vi "Read out IMON.vi"(4 "get more?":bool, 5 "All Channels (T)":bool=TRUE, 7 "Channel":u8, 8 "error in (no error)":errorcluster, 11 "BoardHandle":T2) -> (0 "error out":errorcluster, 1 "IMon constants":T1(array[cluster]), 2 "IMon values (uA)":dbl[](array[numeric]) format="%.2f", 3 "BoardHandle out":T2)   [LabVIEW 2020, in "CAEN PSM.lvlib"]
doc: "This function returns Imon value"
uses:
  CAEN PSM.lvlib
  Private/BoardHandle.ctl
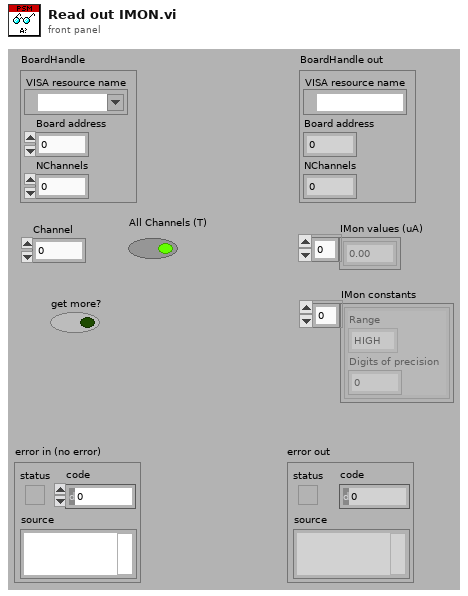
[diagram p1: front panel]
types:
  T1 = cluster{"Range":enum16{"HIGH", "LOW"}, "Digits of precision":i32}[]
  T2 = typedef "CAEN PSM.lvlib/BoardHandle.ctl" = cluster{"VISA resource name":refnum<visa-resource-name>, "Board address":i8, "NChannels":u8}
  T3 = cluster{"Range":enum16{"HIGH", "LOW"}, "Digits of precision":i32}
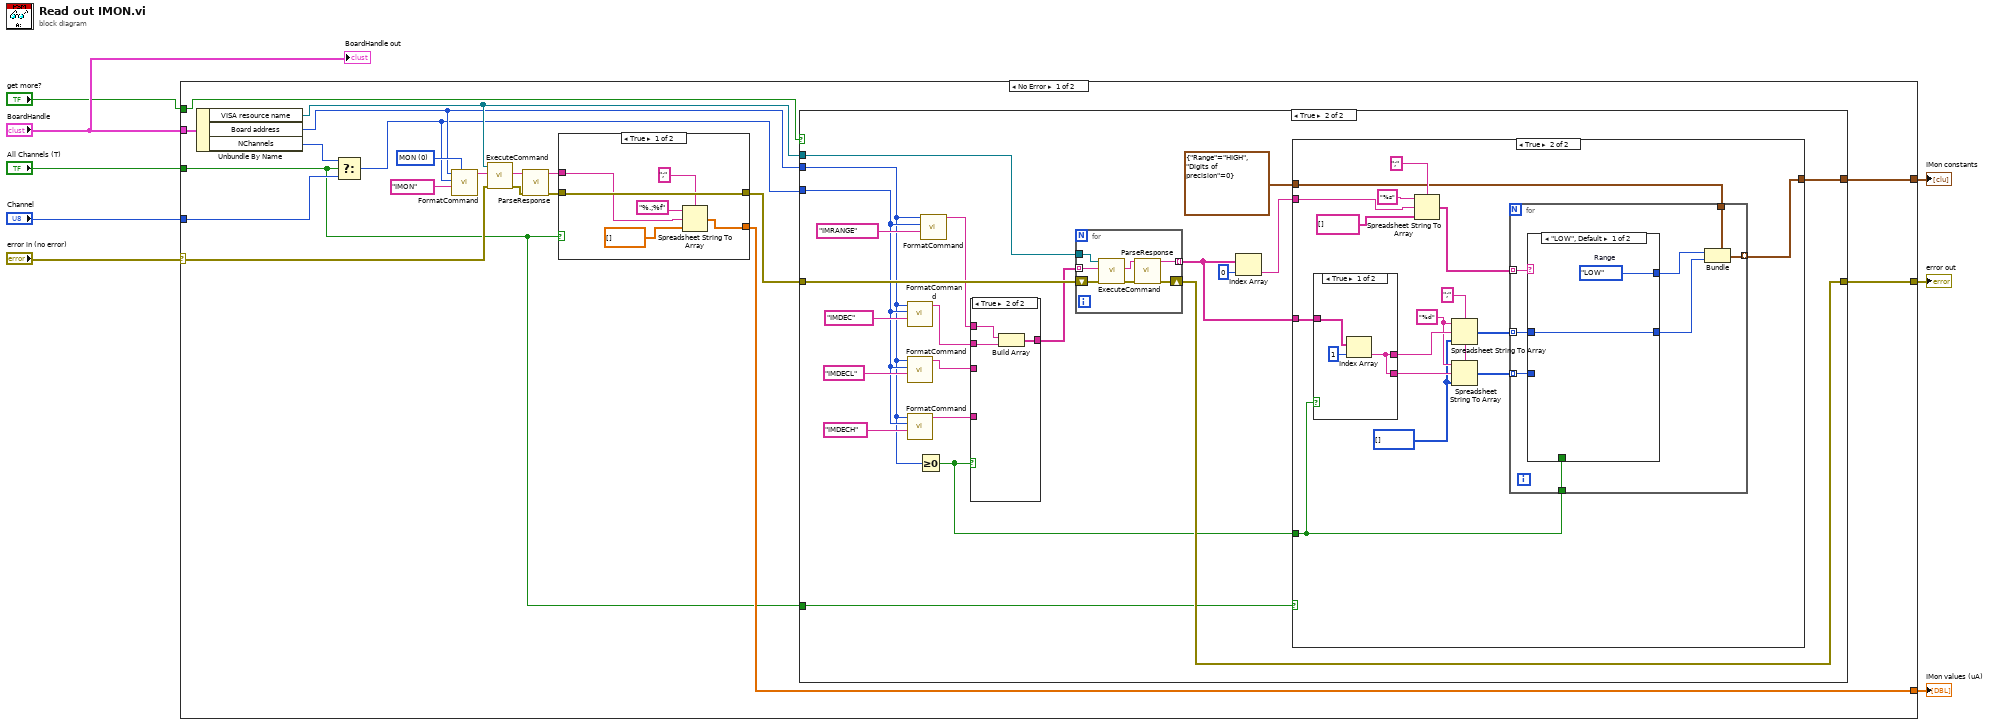
[diagram p0: block diagram]
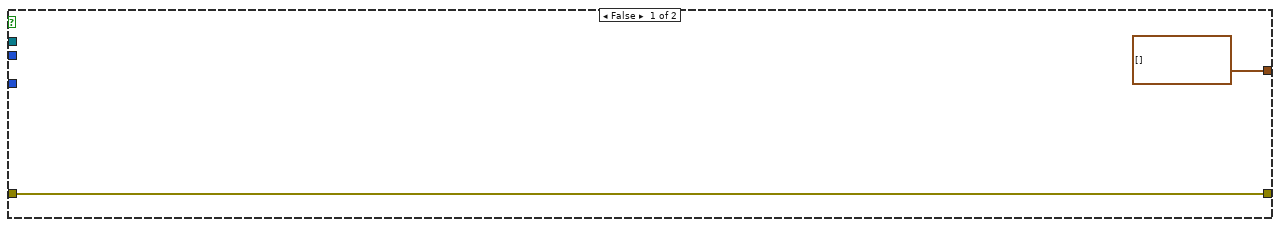
[diagram p2: hidden frame]
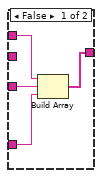
[diagram p3: hidden frame]
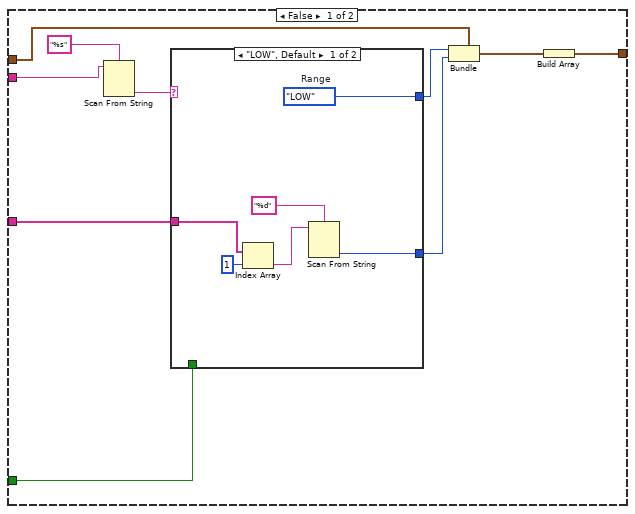
[diagram p4: hidden frame]
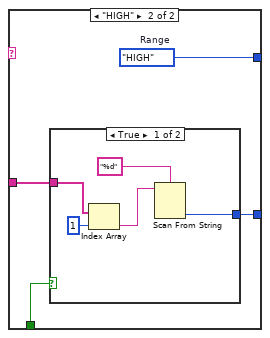
[diagram p5: hidden frame]
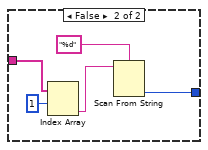
[diagram p6: hidden frame]
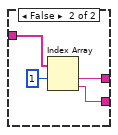
[diagram p7: hidden frame]
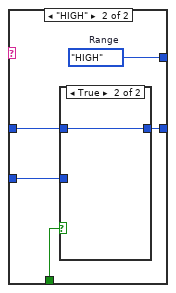
[diagram p8: hidden frame]
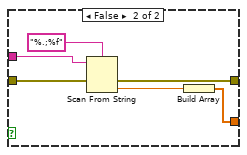
[diagram p10: hidden frame]
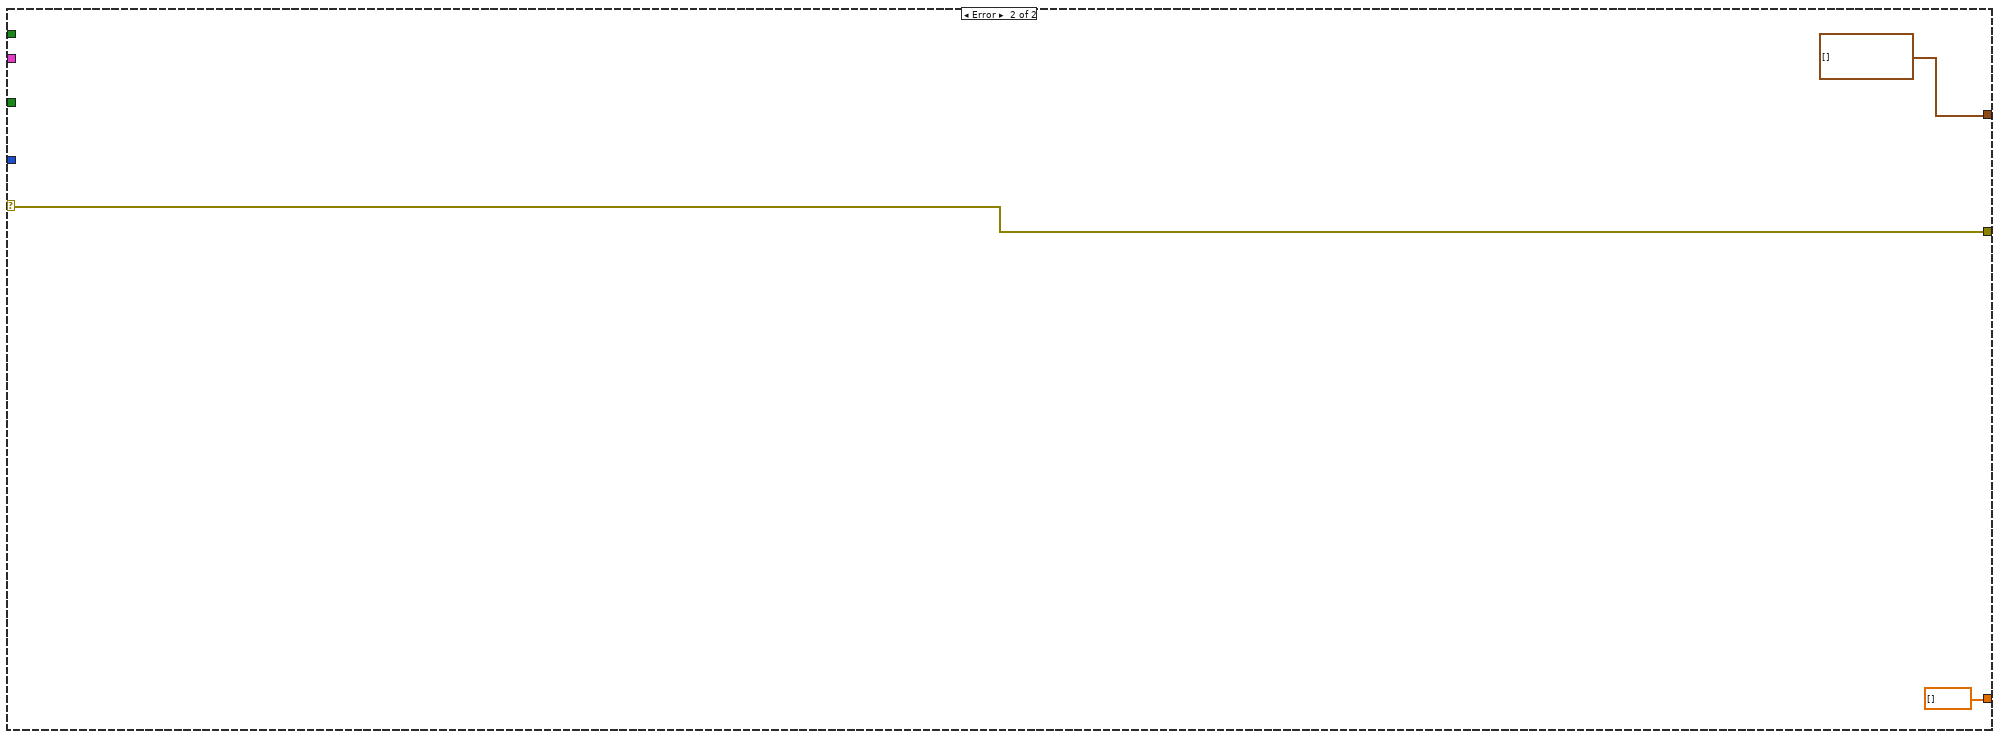
[diagram p11: hidden frame]
diagram:
  n1 = case shown="No Error" "error in (no error)" {
    selector: "error in (no error)" -> [w22 w150]
    tunnel: "All Channels (T)" -> [w9 _]
    tunnel: "Channel" -> [w27 _]
    tunnel: [w11 w150] -> w5
    tunnel: "BoardHandle" -> [w23 _]
    tunnel: [w17 dbl[] [] ("Trip value(s) s")] -> w3
    tunnel: "get more?" -> [w16 _]
    tunnel: [w10 T1 []] -> w1
    frame No Error {
      w28 = u8 0 items=["MON", "SET"] ("CMD")
      n2 = Unbundle By Name(w23) -> ("VISA resource name"=w15:refnum<visa-resource-name>, "Board address"=w14:i8, "NChannels"=w20:u8)
      n3 = Select(t=w20, s=w9, f=w27) -> (s? t:f=w13:u8)
      n4 = call "FormatCommand.vi"("CMD (MON)"=w28, "PAR"="IMON", "CH"=w13, "BD (0)"=w14) -> ("cmd"=w26:string)  [unwired: 7 in]
      n5 = call "ExecuteCommand.vi"("error in (no error)"=w22, "Command"=w26, "VISA resource name"=w15) -> ("error out"=w25:errorcluster, "Response"=w24:string)  [unwired: 6 in, 1 out]
      n6 = call "ParseResponse.vi"("error in (no error)"=w25, "Response"=w24) -> ("error out"=w18:errorcluster, "val"=w19:string)  [unwired: 6 in, 2 out]
      n7 = case shown="True" w9 {
        tunnel: w19 -> [w136 w147]
        tunnel: w18 -> [w141 w145]
        tunnel: [w141 w144] -> w12
        tunnel: [w137 w142] -> w17
        frame True {
          n8 = Spreadsheet String To Array(delimiter (Tab)=";", format string="%.;%f", spreadsheet string=w136, array type (2D Dbl)=dbl[] []) -> (array=w137:dbl[])
        }
        frame False {
          n9 = Scan From String(format string="%.;%f", input string=w147, error in=w145) -> (error out=w144:errorcluster, output 1=w143:dbl)  [unwired: 2 in, 2 out]
          n10 = Build Array(w143) -> (w142:dbl[])
        }
      }
      n11 = case shown="True" w16 {
        tunnel: w12 -> [w30 w48]
        tunnel: [w30 w47] -> w11
        tunnel: w15 -> [_ w49]
        tunnel: w14 -> [_ w35]
        tunnel: w13 -> [_ w41]
        tunnel: [T1 [] w45] -> w10
        tunnel: w9 -> [_ w44]
        frame False {
        }
        frame True {
          n12 = call "FormatCommand.vi"("PAR"="IMDEC", "CH"=w41, "BD (0)"=w35) -> ("cmd"=w40:string)  [unwired: 8 in]
          n13 = call "FormatCommand.vi"("PAR"="IMDECL", "CH"=w41, "BD (0)"=w35) -> ("cmd"=w37:string)  [unwired: 8 in]
          n14 = call "FormatCommand.vi"("PAR"="IMDECH", "CH"=w41, "BD (0)"=w35) -> ("cmd"=w36:string)  [unwired: 8 in]
          n15 = Greater Or Equal To 0?(x=w35) -> (x >= 0?=w32:bool)
          n16 = call "FormatCommand.vi"("PAR"="IMRANGE", "CH"=w41, "BD (0)"=w35) -> ("cmd"=w39:string)  [unwired: 8 in]
          n17 = case shown="True" w32 {
            tunnel: w40 -> [_ w58]
            tunnel: w39 -> [w55 w57]
            tunnel: [w52 w56] -> w38
            tunnel: w37 -> [w54 _]
            tunnel: w36 -> [w53 _]
            frame False {
              n18 = Build Array(w55, w54, w53) -> (w52:string[])
            }
            frame True {
              n19 = Build Array(w57, w58) -> (w56:string[])
            }
          }
          n20 = for {
            tunnel: w38 -> [w135] mode=indexing
            tunnel: w49 -> [w134]
            shift-right: [w132] -> w47
            shift-left: w48 -> [w133]
            tunnel: [w129] -> w31 mode=indexing
            n21 = call "ExecuteCommand.vi"("error in (no error)"=w133, "Command"=w135, "VISA resource name"=w134) -> ("error out"=w131:errorcluster, "Response"=w130:string)  [unwired: 6 in, 1 out]
            n22 = call "ParseResponse.vi"("error in (no error)"=w131, "Response"=w130) -> ("error out"=w132:errorcluster, "val"=w129:string)  [unwired: 6 in, 2 out]
          }
          n23 = Index Array(array=w31, index=0) -> (element=w33:string)
          n24 = case shown="True" w44 {
            tunnel: w33 -> [w68 w100]
            tunnel: T3 {"Range"=enum."HIGH", "Digits of precision"=0} -> [w63 w102]
            tunnel: [w65 w101] -> w45
            tunnel: w32 -> [w60 w89]
            tunnel: w31 -> [w59 w97]
            frame False {
              n25 = Scan From String(format string="%s", input string=w68) -> (output 1=w64:string)  [unwired: 3 in, 3 out]
              n26 = case shown="\"LOW\", Default" w64 {
                tunnel: [w74 w78] -> w62
                tunnel: [w73 w76] -> w61
                tunnel: w60 -> [_ w75]
                tunnel: w59 -> [w72 w77]
                frame "LOW", Default {
                  w74 = enum16{"HIGH", "LOW"}."LOW"  # Range
                  n27 = Index Array(array=w72, index=1) -> (element=w69:string)
                  n28 = Scan From String(format string="%d", input string=w69) -> (output 1=w73:i32)  [unwired: 3 in, 3 out]
                }
                frame "HIGH" {
                  w78 = enum16{"HIGH", "LOW"}."HIGH"  # Range
                  n29 = case shown="True" w75 {
                    tunnel: [w82 w87] -> w76
                    tunnel: w77 -> [w80 w85]
                    frame True {
                      n30 = Index Array(array=w80, index=1) -> (element=w79:string)
                      n31 = Scan From String(format string="%d", input string=w79) -> (output 1=w82:i32)  [unwired: 3 in, 3 out]
                    }
                    frame False {
                      n32 = Index Array(array=w85, index #1=1 ("index")) -> (element #2=w84:string)  [unwired: 1 in, 1 out]
                      n33 = Scan From String(format string="%d", input string=w84) -> (output 1=w87:i32)  [unwired: 3 in, 3 out]
                    }
                  }
                }
              }
              n34 = Bundle(cluster=w63, "Range"=w62, "Digits of precision"=w61) -> (w66:T3)
              n35 = Build Array(w66) -> (w65:T1)
            }
            frame True {
              w93 = ";" ("delimiter (Tab)")
              w94 = "%d" ("format string")
              w92 = i32[] []
              n36 = case shown="True" w89 {
                tunnel: w97 -> [w106 w110]
                tunnel: [w105 w109] -> w96
                tunnel: [w105 w108] -> w95
                frame True {
                  n37 = Index Array(array=w106, index=1) -> (element=w105:string)
                }
                frame False {
                  n38 = Index Array(array=w110, index #1=1 ("index")) -> (element #1=w109:string, element #2=w108:string)  [unwired: 1 in]
                }
              }
              n39 = Spreadsheet String To Array(delimiter (Tab)=";", format string="%s", spreadsheet string=w100, array type (2D Dbl)=string[] []) -> (array=w98:string[])
              n40 = Spreadsheet String To Array(delimiter (Tab)=w93, format string=w94, spreadsheet string=w96, array type (2D Dbl)=w92) -> (array=w91:i32[])
              n41 = Spreadsheet String To Array(delimiter (Tab)=w93, format string=w94, spreadsheet string=w95, array type (2D Dbl)=w92) -> (array=w90:i32[])
              n42 = for {
                tunnel: w102 -> [w119]
                tunnel: [w118] -> w101 mode=indexing
                tunnel: w98 -> [w117] mode=indexing
                tunnel: w91 -> [w115] mode=indexing
                tunnel: w90 -> [w114] mode=indexing
                tunnel: w89 -> [w113]
                n43 = case shown="\"LOW\", Default" w117 {
                  tunnel: [w121 w126] -> w116
                  tunnel: w115 -> [w120 w124]
                  tunnel: w114 -> [_ w122]
                  tunnel: w113 -> [_ w125]
                  tunnel: [w120 w123] -> w112
                  frame "LOW", Default {
                    w121 = enum16{"HIGH", "LOW"}."LOW"  # Range
                  }
                  frame "HIGH" {
                    w126 = enum16{"HIGH", "LOW"}."HIGH"  # Range
                    n44 = case shown="True" w125 {
                      tunnel: [w127 w128] -> w123
                      tunnel: w124 -> [_ w128]
                      tunnel: w122 -> [w127 _]
                      frame False {
                      }
                      frame True {
                      }
                    }
                  }
                }
                n45 = Bundle(cluster=w119, "Range"=w116, "Digits of precision"=w112) -> (w118:T3)
              }
            }
          }
        }
      }
    }
    frame Error {
    }
  }
  "error out" <- w5
  "IMon values (uA)" <- w3
  "IMon constants" <- w1
  "BoardHandle out" <- "BoardHandle"
